vi "Get PGI List.vi"(0 "pgiType":i32, 1 "piNumListItems":i32, 5 "piDevNumList":i32, 7 "ppszIPList":string, 9 "ppszMACList":string, 11 "error in (no error)":errorcluster caption="错误输入（无错误）") -> (3 "piNumListItems out":i32, 4 "function return":i32, 6 "piDevNumList out":i32, 8 "ppszIPList out":string, 10 "ppszMACList out":string, 15 "error out":errorcluster caption="错误输出")   [LabVIEW 2018]
doc: "extern int __stdcall APSxGetPGIList (int pgiType, int *piDevNumList, char **ppszIPList, char **ppszMACList, int *piNumListItems);"
uses:
  APSx.dll/APSx.dll
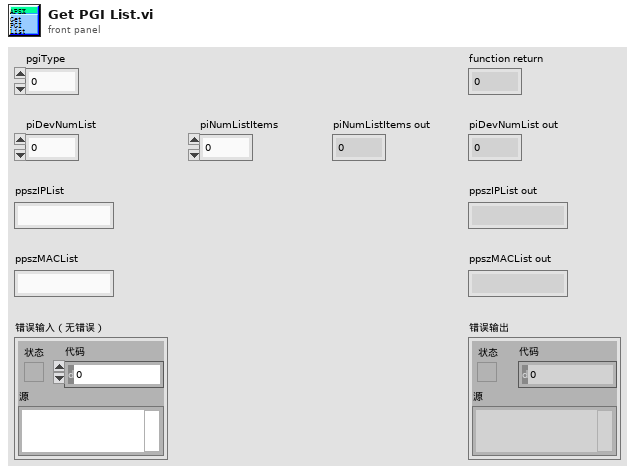
[diagram p1: front panel]
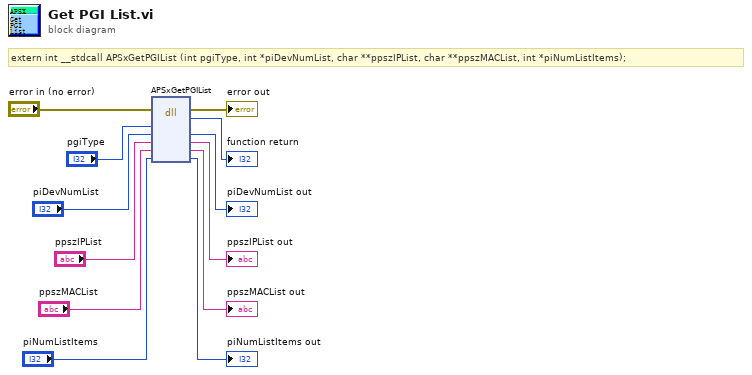
[diagram p0: block diagram]
diagram:
  # "extern int __stdcall APSxGetPGIList (int pgiType, int *piDevNumList, char **ppszIPList, char **ppszMACList, int *piNumListItems);"
  n1 = dll-call lib="PTH2[abs D项目Feng恒隆项目Labview传感器对中台SourcesAPSx.dllAPSx.*" fn="APSxGetPGIList"(error in="error in (no error)", "pgiType"="pgiType", "piDevNumList"="piDevNumList", "ppszIPList"="ppszIPList", "ppszMACList"="ppszMACList", "piNumListItems"="piNumListItems") -> (error out=→"error out":errorcluster, →"function return":i32, "piDevNumList"=→"piDevNumList out":i32, "ppszIPList"=→"ppszIPList out":string, "ppszMACList"=→"ppszMACList out":string, "piNumListItems"=→"piNumListItems out":i32)  [unwired: 3 in, 1 out]
